vi "getWavelength.vi"(4 "Fiber Num":i32, 6 "Error":bool, 7 "VISA resource name":refnum<visa-resource-name>="ASRL13::INSTR") -> (0 "Wavelength":u32, 2 "Error":bool, 3 "dup VISA resource name":refnum<visa-resource-name>="ASRL13::INSTR")   [LabVIEW 2020, in "Library Instrument & Equipement.lvlib" / "Library LED Analyser.lvlib"]
uses:
  Library LED Analyser.lvlib
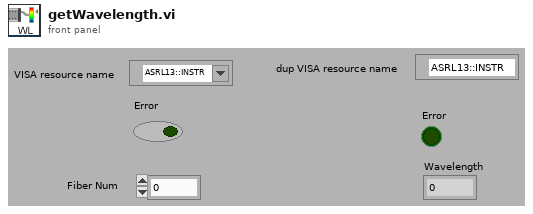
[diagram p1: front panel]
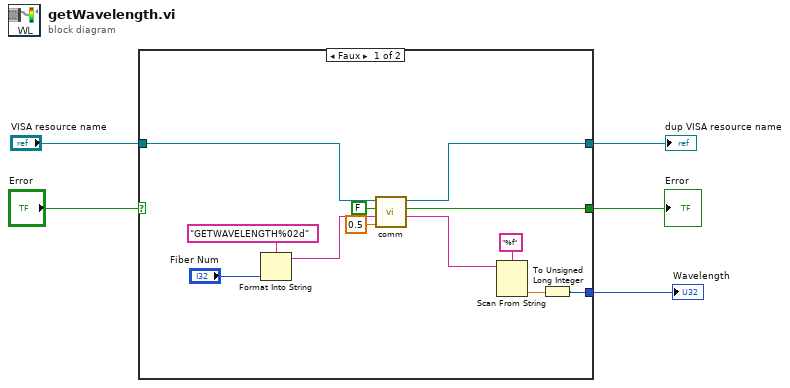
[diagram p0: block diagram]
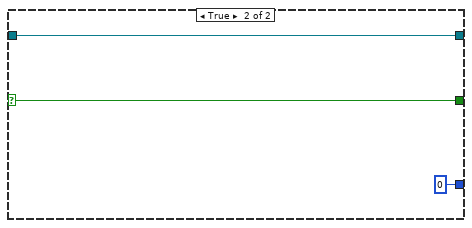
[diagram p2: hidden frame]
diagram:
  n1 = case shown="Faux" "Error" {
    selector: "Error" -> [_ w20]
    tunnel: "VISA resource name" -> [w17 w19]
    tunnel: [w11 w20] -> w4
    tunnel: [w10 w19] -> w3
    tunnel: [w8 u32 0] -> w1
    frame False {
      n2 = Format Into String(format string="GETWAVELENGTH%02d" ("Substring"), "Fiber Num") -> (resulting string=w14:string)  [unwired: 2 in, 1 out]
      n3 = call "comm.vi"("Timeout (s)"=0.5, "Command"=w14, "Error"=FALSE, "VISA resource name"=w17) -> ("Response"=w12:string, "Error"=w11:bool, "dup VISA resource name"=w10:refnum<visa-resource-name>)  [unwired: 2 in, 1 out]
      n4 = Scan From String(format string="%f", input string=w12) -> (output 1=w9:dbl)  [unwired: 3 in, 3 out]
      n5 = To Unsigned Long Integer(number=w9) -> (unsigned 32bit integer=w8:u32)
    }
    frame True {
    }
  }
  "Wavelength" <- w1
  "Error" <- w4
  "dup VISA resource name" <- w3
